vi "mergeError.vi"(8 "error in (no error)":errorcluster, 11 "error in (no error) 2":errorcluster) -> (0 "error out":errorcluster)   [LabVIEW 2014, in "FH 55.lvlib"]
uses:
  FH 55.lvlib
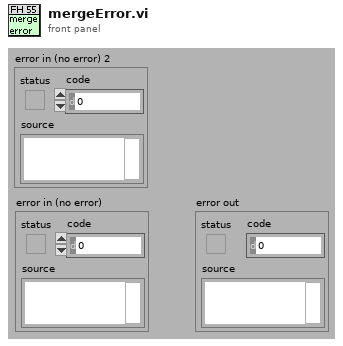
[diagram p1: front panel]
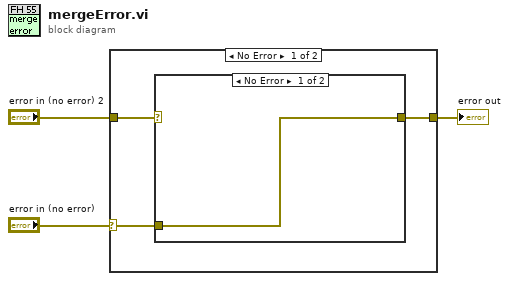
[diagram p0: block diagram]
diagram:
  n1 = case shown="No Error" "error in (no error)" {
    selector: "error in (no error)" -> [w4 w9]
    tunnel: "error in (no error) 2" -> [w6 _]
    tunnel: [w5 w9] -> w3
    frame No Error {
      n2 = case shown="No Error" w6 {
        selector: w6 -> [_ w8]
        tunnel: [w7 w8] -> w5
        tunnel: w4 -> [w7 _]
        frame No Error {
        }
        frame Error {
        }
      }
    }
    frame Error {
    }
  }
  "error out" <- w3
